vi "create Timings.vi"(8 "error in (no error)":errorcluster, 10 "Parameters":u32[](array[numeric]), 11 "Spannungseinbruch in":refnum<class "Spannungseinbruch.lvclass">) -> (0 "error out":errorcluster, 1 "wait":i32[](array[numeric])=[0, 30000, 0, 0], 2 "timeout":u32[](array[numeric]), 3 "Spannungseinbruch out":refnum<class "Spannungseinbruch.lvclass">)   [LabVIEW 2013, in "Spannungseinbruch.lvclass"]
uses:
  Spannungseinbruch.lvclass
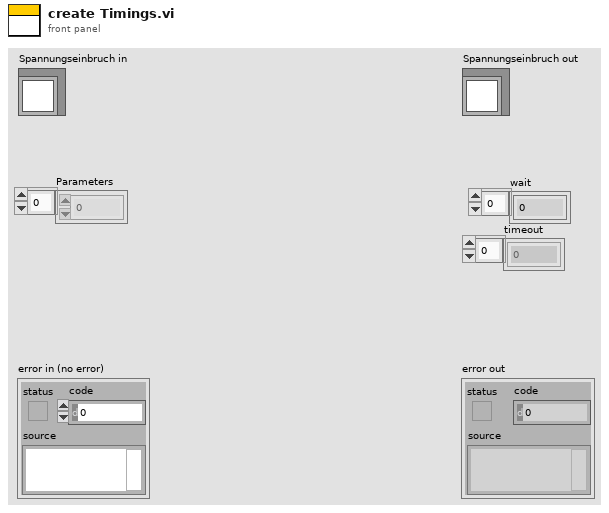
[diagram p1: front panel]
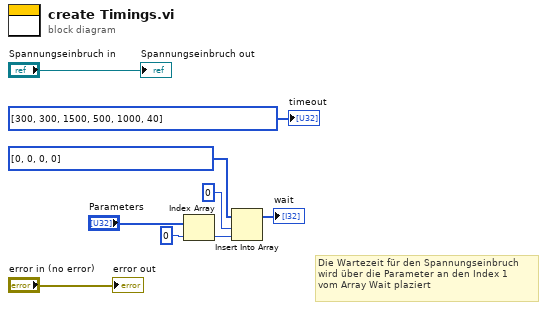
[diagram p0: block diagram]
diagram:
  # "Die Wartezeit für den Spannungseinbruch\nwird über die Parameter an den Index 1\nvom Array Wait plaziert"
  n1 = Index Array(array="Parameters", index=0) -> (element=w4:u32)
  n2 = Insert Into Array(array=i32[] [0, 0, 0, 0] ("Timings"), index=0, new element=w4) -> (→"wait":i32[])
  "error out" <- "error in (no error)"
  "Spannungseinbruch out" <- "Spannungseinbruch in"
  "timeout" <- i32[] [300, 300, 1500, 500, 1000, 40] ("Timings")
